vi "RunEventAndMonitor.vi"(8 "error in (no error)":errorcluster, 10 "Estimated Time (ms)":u32, 11 "Asylum_Driver in":refnum<class "Asylum_Driver.lvclass">) -> (0 "error out":errorcluster, 3 "Asylum_Driver out":refnum<class "Asylum_Driver.lvclass">)   [LabVIEW 2019, in "Asylum_Driver.lvclass"]
uses:
  Asylum_Driver.lvclass
  AFM Driver/AFM_Driver.lvclass
  C:/Users/Albro/Documents/GitHub/AFM-Lithography/lvsrc/AFMs/AFM Driver/AFM_Driver.lvclass
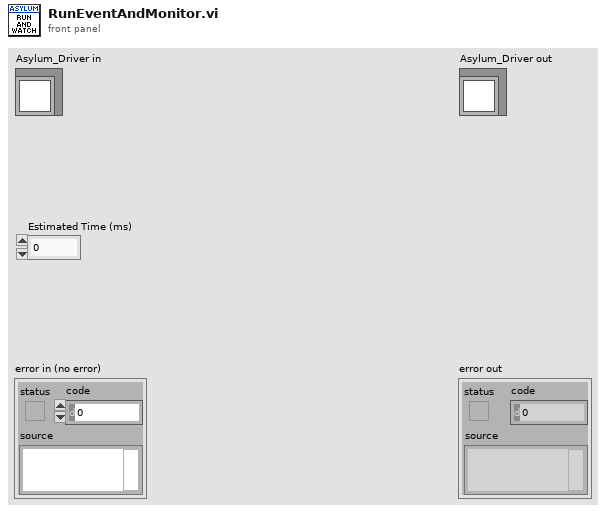
[diagram p1: front panel]
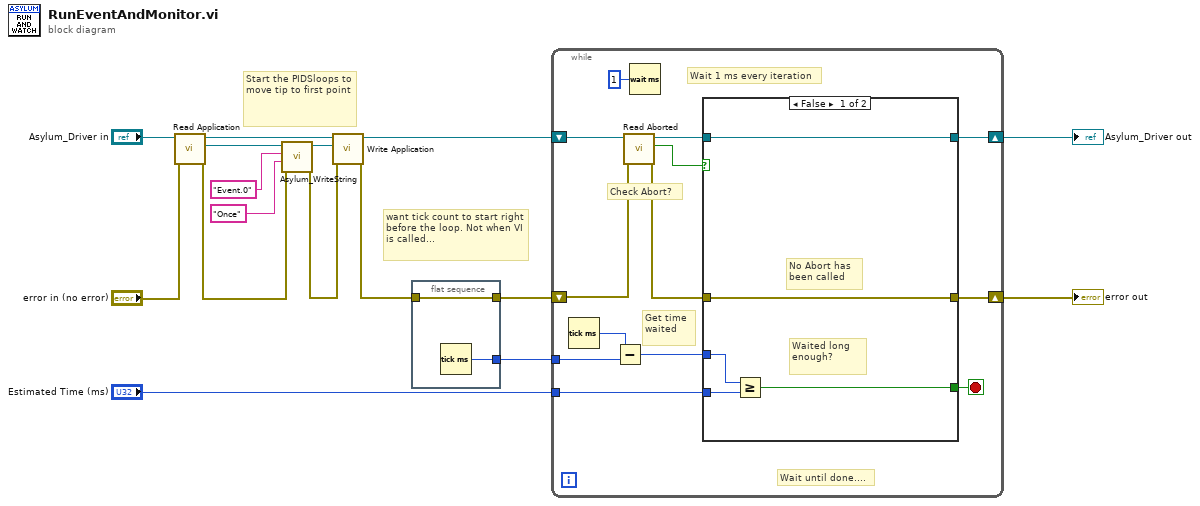
[diagram p0: block diagram]
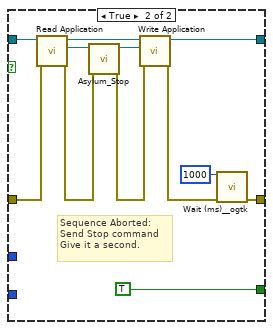
[diagram p2: hidden frame]
diagram:
  # "want tick count to start right before the loop. Not when VI is called..."
  # "Start the PIDSloops to move tip to first point"
  n1 = call-dynamic "Read Application.vi"("error in (no error)"="error in (no error)", "Asylum_Driver in"="Asylum_Driver in") -> ("error out"=w3:errorcluster, "Application"=w5:refnum<k7>, "Asylum_Driver out"=w6:refnum<class "Asylum_Driver.lvclass">)  [unwired: 7 in]
  n2 = call <userlib>:"Asylum_WriteString.vi"("error in (no error)"=w3, "valueString"="Once", "parameterName"="Event.0", "Application"=w5) -> ("error out"=w2:errorcluster, "Application"=w8:refnum<k7>)  [unwired: 6 in]
  n3 = call-dynamic "Write Application.vi"("error in (no error)"=w2, "Application"=w8, "Asylum_Driver in"=w6) -> ("error out"=w1:errorcluster, "Asylum_Driver out"=w9:refnum<class "Asylum_Driver.lvclass">)  [unwired: 7 in]
  n4 = flat-sequence {
    tunnel: [w17] -> w12
    tunnel: w1 -> [w18]
    tunnel: [w18] -> w13
    frame #0 {
      n5 = Tick Count (ms)() -> (millisecond timer value=w17:u32)
    }
  }
  n6 = while {
    shift-right: [w31] -> w11
    shift-left: w13 -> [w23]
    tunnel: w12 -> [w28]
    tunnel: "Estimated Time (ms)" -> [w25]
    shift-right: [w19] -> w10
    shift-left: w9 -> [w24]
    stop <- w30 stop-if-true
    # "Wait until done...."
    # "Check Abort?"
    # "Wait 1 ms every iteration"
    # "Get time waited"
    n7 = Tick Count (ms)() -> (millisecond timer value=w29:u32)
    n8 = Subtract(x=w29, y=w28) -> (x-y=w26:u32)
    n9 = call "Read Aborted.vi"("error in (no error)"=w23, "AFM_Driver in"=w24) -> ("error out"=w22:errorcluster, "Aborted?"=w21:bool, "AFM_Driver out"=w20:refnum<class "Asylum_Driver.lvclass">)  [unwired: 7 in]
    n10 = Wait (ms)(milliseconds to wait=u32 1) -> ()  [unwired: 1 out]
    n11 = case shown="False" w21 {
      tunnel: w22 -> [w36 w37]
      tunnel: [w36 w47] -> w31
      tunnel: [w33 TRUE] -> w30
      tunnel: w26 -> [w35 _]
      tunnel: w25 -> [w34 _]
      tunnel: w20 -> [w32 w45]
      tunnel: [w32 w41] -> w19
      frame False {
        # "No Abort has been called"
        # "Waited long enough?"
        n12 = Greater Or Equal?(x=w35, y=w34) -> (x >= y?=w33:bool)
      }
      frame True {
        # "Sequence Aborted:\nSend Stop command\nGive it a second."
        n13 = call-dynamic "Read Application.vi"("error in (no error)"=w37, "Asylum_Driver in"=w45) -> ("error out"=w38:errorcluster, "Application"=w44:refnum<k7>, "Asylum_Driver out"=w42:refnum<class "Asylum_Driver.lvclass">)  [unwired: 7 in]
        n14 = call <userlib>:"Asylum_Stop.vi"("error in (no error)"=w38, "Application"=w44) -> ("error out"=w40:errorcluster, "Application"=w43:refnum<k7>)  [unwired: 8 in]
        n15 = call-dynamic "Write Application.vi"("error in (no error)"=w40, "Application"=w43, "Asylum_Driver in"=w42) -> ("error out"=w39:errorcluster, "Asylum_Driver out"=w41:refnum<class "Asylum_Driver.lvclass">)  [unwired: 7 in]
        n16 = call <userlib>:"Wait (ms)__ogtk.vi"("error in (no error)"=w39, "milliseconds to wait"=u32 1000) -> ("error out"=w47:errorcluster)  [unwired: 8 in, 1 out]
      }
    }
  }
  "error out" <- w11
  "Asylum_Driver out" <- w10
